vi "Create ooDocument.vi"(8 "error in (no error)":errorcluster, 9 "Document":refnum<k24>, 11 "ooDocument in":refnum<class "ooDocument.lvclass">) -> (0 "error out":errorcluster, 3 "ooDocument out":refnum<class "ooDocument.lvclass">)   [LabVIEW 2009, in "ooDocument.lvclass"]
uses:
  ooDocument.lvclass
  C:/Projets/LAVAG/OpenOfficeRGT/AODL/DLLs/AODL.dll
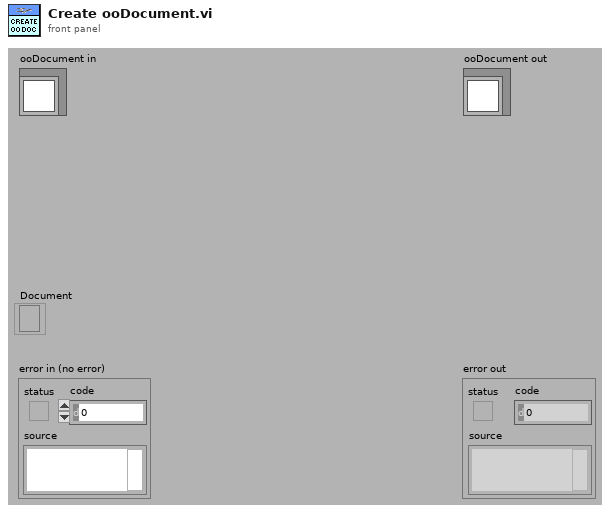
[diagram p1: front panel]
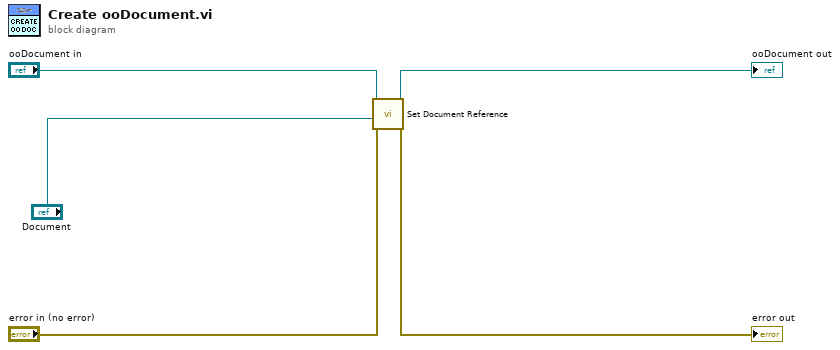
[diagram p0: block diagram]
diagram:
  n1 = call "Set Document Reference.vi"("error in (no error)"="error in (no error)", "Document"="Document", "ooDocument in"="ooDocument in") -> ("error out"=→"error out":errorcluster, "ooDocument out"=→"ooDocument out":refnum<class "ooDocument.lvclass">)  [unwired: 7 in]
